vi "M100HoldLot.vi"() -> ()   [LabVIEW 2012]
uses:
  <vilib>/addons/database/Auxilliary.llb/DB Tools Cursor Type.ctl
  <vilib>/Utility/NIReport.llb/NI_report.lvclass
  <vilib>/addons/database/Connection.llb/DB Tools Open Connec (Path).vi
  <vilib>/addons/database/Connection.llb/Conn Execute.vi
  <vilib>/addons/database/Recordset.llb/Rec Fetch Recordset Data (R).vi
  <vilib>/addons/database/Recordset.llb/Rec Destroy - Connection.vi
  <vilib>/addons/database/_DB Variant To Data/Database Variant To Data.xnode
  <vilib>/Utility/NIReport.llb/Excel/NI_Excel.lvclass
  <vilib>/addons/database/NI_Database_API.lvlib
  <vilib>/Utility/SMTP/NI_SMTPEmail.lvlib
panel:
  out "error out 2":errorcluster
  in  "MIME content-type (application/octet-stream)":string="application/octet-stream"
  out "error out 3":errorcluster
  in  "template (empty)":path=path "O:/Monitor/Report/Hold Lot Repor.xls"
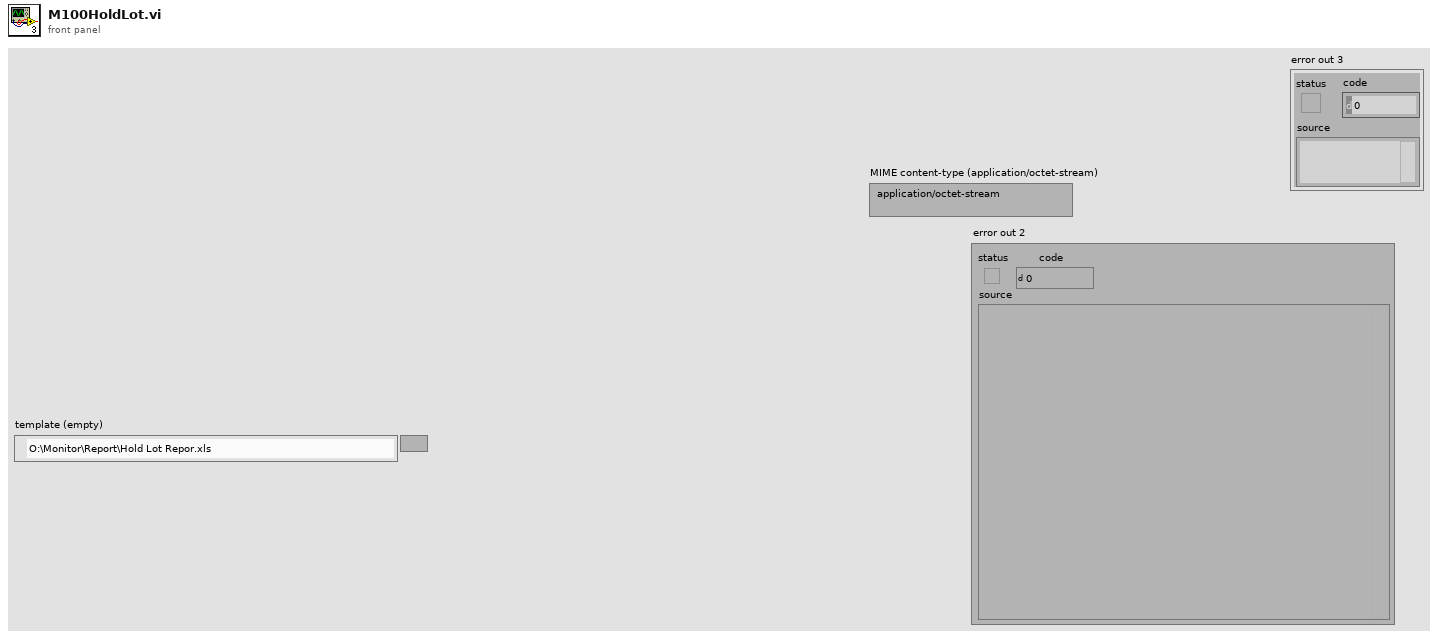
[diagram p1: front panel]
types:
  T1 = typedef "NI_Database_API.lvlib/DB Tools Cursor Type.ctl" = enum16{"forward-only", "keyset", "dynamic", "static"}
  T2 = enum16{"Standard Report", "HTML", "Word", "Excel"}
  T3 = typedef "NI_Database_API.lvlib/Conn ObjectReference.ctl" = refnum<k1>
  T4 = typedef "NI_Database_API.lvlib/Rec ObjectReference.ctl" = refnum<k1>
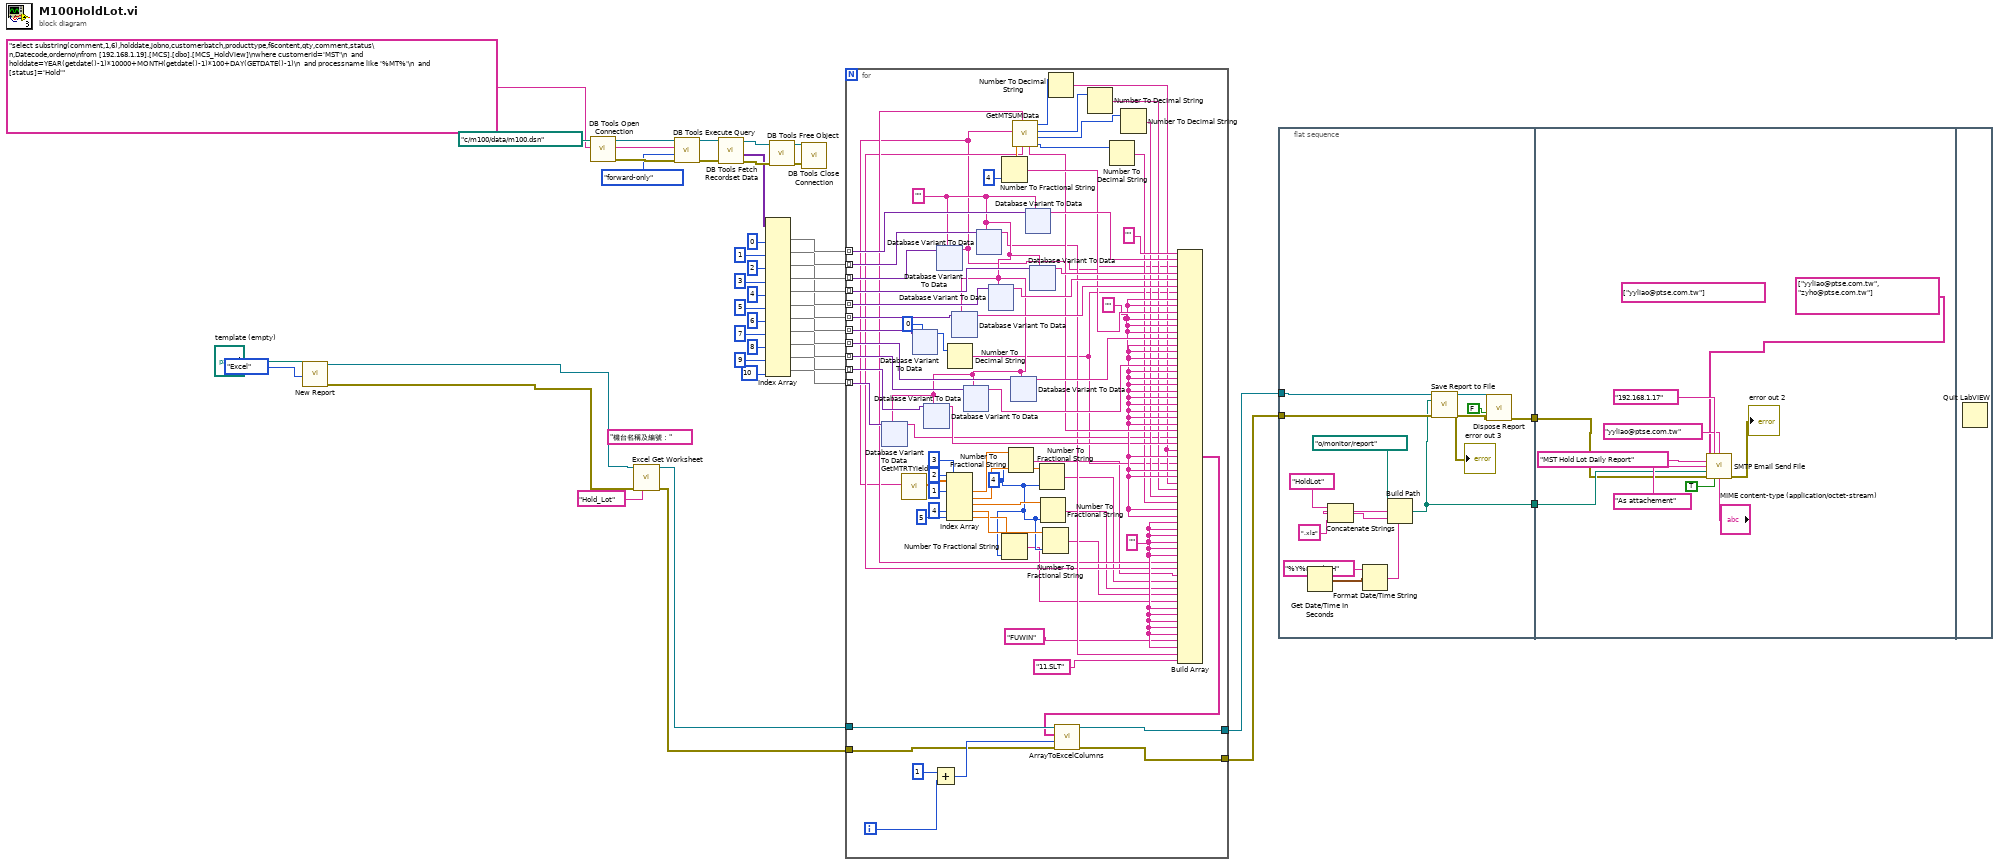
[diagram p0: block diagram]
diagram:
  (unwired) "機台名稱及編號：" ("formula")
  n1 = call <vilib>:"New Report.vi"("report type"=T2."Excel" ("Report Type"), "template (empty)"="template (empty)") -> ("report out"=w44:refnum<class "NI_report.lvclass">, "error out"=w43:errorcluster)  [unwired: 12 in]
  n2 = call-poly <vilib>:"DB Tools Open Connection.vi"("connection information"=path "c:/m100/data/m100.dsn") -> ("error out"=w38:errorcluster, "connection reference"=w39:T3)  [unwired: 7 in]
  n3 = call <vilib>:"Excel Get Worksheet.vi"("report in"=w44, "error in (no error)"=w43, "name (\"\")"="Hold_Lot" ("name (\"\")")) -> ("report out"=w10:refnum<class "NI_report.lvclass">, "error out"=w9:errorcluster)  [unwired: 11 in]
  n4 = call-poly <vilib>:"DB Tools Execute Query.vi"("error in (no error)"=w38, "cursor type"=DB_Tools_Cursor_Type."forward-only", "SQL query"="select substring(comment,1,6),holddate,jobno,customerbatch,producttype,f6content,qty,comment,status\n,Datecode,orderno\nfrom [192.168.1.19].[MCS].[dbo].[MCS_HoldView]\nwhere customerid='MST'\n  and holddate=YEAR(getdate()-1)*10000+MONTH(getdate()-1)*100+DAY(GETDATE()-1)\n  and processname like '%MT%'\n  and [status]='Hold'", "connection reference"=w39) -> ("error out"=w37:errorcluster, "recordset reference"=w36:T4)  [unwired: 4 in]
  n5 = call-poly <vilib>:"DB Tools Fetch Recordset Data.vi"("error in (no error)"=w37, "recordset reference"=w36) -> ("error out"=w31:errorcluster, "recordset data"=w29:variant[][], "recordset reference out"=w33:T4)  [unwired: 3 in]
  n6 = Index Array(array=w29, index (col) #1=0 ("disabled index (col)"), index (col) #2=1 ("index (col)"), index (col) #3=2 ("index (col)"), index (col) #4=3 ("index (col)"), index (col) #5=4 ("index (col)"), index (col) #6=5 ("index (col)"), index (col) #7=6 ("index (col)"), index (col) #8=7 ("index (col)"), index (col) #9=8 ("index (col)"), index (col) #10=9 ("index (col)"), index (col) #11=10 ("index (col)")) -> (element #1=w19:variant[], element #2=w18:variant[], element #3=w17:variant[], element #4=w16:variant[], element #5=w15:variant[], element #6=w14:variant[], element #7=w13:variant[], element #8=w12:variant[], element #9=w11:variant[], element #10=w6:variant[], element #11=w5:variant[])  [unwired: 11 in]
  n7 = call-poly <vilib>:"DB Tools Free Object.vi"("error in (no error)"=w31, "recordset reference"=w33) -> ("error out"=w30:errorcluster, "connection reference"=w32:T3)  [unwired: 8 in]
  n8 = call <vilib>:"DB Tools Close Connection.vi"("error in (no error)"=w30, "connection reference"=w32) -> ()  [unwired: 5 in, 1 out]
  n9 = for {
    tunnel: w19 -> [w114] mode=indexing
    tunnel: w18 -> [w113] mode=indexing
    tunnel: w17 -> [w112] mode=indexing
    tunnel: w16 -> [w111] mode=indexing
    tunnel: w15 -> [w110] mode=indexing
    tunnel: w14 -> [w109] mode=indexing
    tunnel: w13 -> [w108] mode=indexing
    tunnel: w12 -> [w107] mode=indexing
    tunnel: w11 -> [w106] mode=indexing
    tunnel: w10 -> [w97]
    tunnel: w9 -> [w96]
    tunnel: w6 -> [w90] mode=indexing
    tunnel: w5 -> [w89] mode=indexing
    tunnel: [w87] -> w2
    tunnel: [w86] -> w1
    i -> [w98]
    w56 = i16 4 ("precision (6)")
    w70 = ""
    w80 = ""
    w88 = ""
    n10 = xnode "Database Variant To Data"("database variant"=w89, "type"=w88) -> ("data"=w73:string)  [unwired: 1 in, 1 out]
    n11 = xnode "Database Variant To Data"("database variant"=w108, "type"=0) -> ("data"=w104:i32)  [unwired: 1 in, 1 out]
    n12 = xnode "Database Variant To Data"("database variant"=w90, "type"=w88) -> ("data"=w79:string)  [unwired: 1 in, 1 out]
    n13 = Add(x=1, y=w98) -> (x+y=w99:i32)
    n14 = xnode "Database Variant To Data"("database variant"=w112, "type"=w88) -> ("data"=w63:string)  [unwired: 1 in, 1 out]
    n15 = call "GetMTRTYield.vi"("RCNO"=w63) -> ("Array"=w62:dbl[])  [unwired: 10 in]
    n16 = Index Array(array=w62, index #1=1 ("index"), index #2=2 ("index"), index #3=3 ("index"), index #4=4 ("index"), index #5=5 ("index")) -> (element #1=w61:dbl, element #2=w60:dbl, element #3=w59:dbl, element #4=w58:dbl, element #5=w57:dbl)
    n17 = Number To Decimal String(number=w104) -> (decimal integer string=w66:string)  [unwired: 1 in]
    n18 = xnode "Database Variant To Data"("database variant"=w109, "type"=w88) -> ("data"=w101:string)  [unwired: 1 in, 1 out]
    n19 = xnode "Database Variant To Data"("database variant"=w106, "type"=w88) -> ("data"=w92:string)  [unwired: 1 in, 1 out]
    n20 = xnode "Database Variant To Data"("database variant"=w113, "type"=w88) -> ("data"=w69:string)  [unwired: 1 in, 1 out]
    n21 = xnode "Database Variant To Data"("database variant"=w110, "type"=w88) -> ("data"=w102:string)  [unwired: 1 in, 1 out]
    n22 = Number To Fractional String(number=w57, precision (6)=w56) -> (F-format string=w46:string)  [unwired: 2 in]
    n23 = Number To Fractional String(number=w61, precision (6)=w56) -> (F-format string=w50:string)  [unwired: 2 in]
    n24 = xnode "Database Variant To Data"("database variant"=w107, "type"=w88) -> ("data"=w91:string)  [unwired: 1 in, 1 out]
    n25 = call "GetMTSUMData.vi"("RCNO"=w63) -> ("bin4"=w74:i32, "bin3"=w76:i32, "bin2"=w78:i32, "bin1"=w82:i32, "Program"=w81:string, "EndDate"=w64:string, "StartDate"=w65:string, "Yield"=w85:dbl)  [unwired: 2 in, 1 out]
    n26 = Number To Fractional String(number=w85, precision (6)=i16 4) -> (F-format string=w83:string)  [unwired: 2 in]
    n27 = xnode "Database Variant To Data"("database variant"=w114, "type"=w88) -> ("data"=w94:string)  [unwired: 1 in, 1 out]
    n28 = xnode "Database Variant To Data"("database variant"=w111, "type"=w88) -> ("data"=w103:string)  [unwired: 1 in, 1 out]
    n29 = Number To Fractional String(number=w60, precision (6)=w56) -> (F-format string=w49:string)  [unwired: 2 in]
    n30 = Number To Fractional String(number=w59, precision (6)=w56) -> (F-format string=w48:string)  [unwired: 2 in]
    n31 = Number To Fractional String(number=w58, precision (6)=w56) -> (F-format string=w47:string)  [unwired: 2 in]
    n32 = Number To Decimal String(number=w82) -> (decimal integer string=w71:string)  [unwired: 1 in]
    n33 = Number To Decimal String(number=w78) -> (decimal integer string=w77:string)  [unwired: 1 in]
    n34 = Number To Decimal String(number=w74) -> (decimal integer string=w72:string)  [unwired: 1 in]
    n35 = Number To Decimal String(number=w76) -> (decimal integer string=w75:string)  [unwired: 1 in]
    n36 = Build Array("" ("element"), w94, w63, w103, w102, w101, w66, w80, w80, w83, w80, w80, w80, w91, w80, w80, w80, w92, w80, w80, w80, w80, w80, w80, w80, w80, w80, w81, w73, w79, w71, w80, w66, w80, w80, w71, w77, w75, w72, w80, w80, w70, w70, w70, w70, w70, w70, w65, w64, w50, w49, w48, w47, w46, w70, w70, w70, w70, w70, "FUWIN", w70, w69, "11.SLT") -> (w95:string[])
    n37 = call "ArrayToExcelColumns.vi"("error in (no error)"=w96, "start row"=w99, "ArrayData"=w95, "report in"=w97) -> ("error in (no error) 2"=w86:errorcluster, "report in 2"=w87:refnum<class "NI_report.lvclass">)  [unwired: 6 in]
  }
  n38 = flat-sequence {
    tunnel: w2 -> [w476]
    tunnel: w1 -> [w475]
    tunnel: [w469] -> w4
    tunnel: [w468] -> w3
    tunnel: w4 -> [w482]
    tunnel: w3 -> [w483]
    frame #0 {
      n39 = Get Date/Time In Seconds() -> (seconds since 1Jan1904=w472:timestamp)
      n40 = Format Date/Time String(time format string (%c)="%Y%m%d%H", seconds (now)=w472) -> (date/time string=w470:string)  [unwired: 1 in]
      n41 = Concatenate Strings("HoldLot" ("string"), w470, ".xls" ("string")) -> (w477:string)
      n42 = Build Path(base path=path "o:/monitor/report", name or relative path=w477) -> (appended path=w468:path)
      n43 = call-dynamic "Save Report to File.vi"("report in"=w476, "report file path"=w468, "error in (no error)"=w475) -> ("report out"=w479:refnum<class "NI_report.lvclass">, "error out"=w478:errorcluster)  [unwired: 11 in]
      "error out 3" <- w478
      n44 = call-dynamic "Dispose Report.vi"("report in"=w479, "save changes? (F)"=FALSE, "error in (no error)"=w478) -> ("error out"=w469:errorcluster)  [unwired: 12 in]
    }
    frame #1 {
      (unwired) string[] ["yyliao@ptse.com.tw"] ("recipients")
      n45 = call <vilib>:"SMTP Email Send File.vi"("recipients"=string[] ["yyliao@ptse.com.tw", "zyho@ptse.com.tw"], "mail server"="192.168.1.17", "return address"="yyliao@ptse.com.tw", "subject ([No Subject])"="MST Hold Lot Daily Report", "message"="As attachement", "file path"=w483, "error in (no error)"=w482, "binary? (F)"=TRUE, "MIME content-type (application/octet-stream)"="MIME content-type (application/octet-stream)") -> ("error out"=→"error out 2":errorcluster)  [unwired: 5 in, 1 out]
    }
    frame #2 {
      n46 = Quit LabVIEW() -> ()  [unwired: 1 in]
    }
  }
